vi "Format CSV.vi"(8 "error in (no error)":errorcluster, 9 "delimiter":string=",", 10 "CSV File Input":path, 11 "Original CSV Format":enum16{"Format A", "Format B"}(ring)) -> (0 "error out":errorcluster, 1 "Parcel Length":i32[](array[numeric]), 2 "All Terminal Data":T1(array[cluster]))   [LabVIEW 2017] (continued)
"28:39.7", "28:39.8", "28:39.8", "28:39.8", "28:39.9", "28:39.9", "28:39.9", "28:40.0", "28:40.0", "28:40.0", "28:40.1", "28:40.1", "28:40.1", "28:40.2", "28:40.2", "28:40.2", "28:40.3", "28:40.3", "28:40.3", "28:40.4", "28:40.4", "28:40.4", "28:40.5", "28:40.5", "28:40.5", "28:40.6", "28:40.6", "28:40.6", "28:40.7", "28:40.7", "28:40.7", "28:40.8", "28:40.8", "28:40.8", "28:40.9", "28:40.9", "28:40.9", "28:41.0", "28:41.0", "28:41.0", "28:41.1", "28:41.1", "28:41.1", "28:41.2", "28:41.2", "28:41.2", "28:41.3", "28:41.3", "28:41.3", "28:41.4", "28:41.4", "28:41.4", "28:41.5", "28:41.5", "28:41.5", "28:41.6", "28:41.6", "28:41.6", "28:41.7", "28:41.7", "28:41.7", "28:41.8", "28:41.8", "28:41.8", "28:41.9", "28:41.9", "28:41.9", "28:42.0", "28:42.0", "28:42.0", "28:42.1", "28:42.1", "28:42.1", "28:42.2", "28:42.2", "28:42.2", "28:42.3", "28:42.3", "28:42.3", "28:42.4", "28:42.4", "28:42.4", "28:42.5", "28:42.5", "28:42.5", "28:42.6", "28:42.6", "28:42.6", "28:42.7", "28:42.7", "28:42.7", "28:42.8", "28:42.8", "28:42.8", "28:42.9", "28:42.9", "28:42.9", "28:43.0", "28:43.0", "28:43.0", "28:43.1", "28:43.1", "28:43.1", "28:43.2", "28:43.2", "28:43.2", "28:43.3", "28:43.3", "28:43.3", "28:43.4", "28:43.4", "28:43.4", "28:43.5", "28:43.5", "28:43.5", "28:43.6", "28:43.6", "28:43.6", "28:43.7", "28:43.7", "28:43.7", "28:43.8", "28:43.8", "28:43.8", "28:43.9", "28:43.9", "28:43.9", "28:44.0", "28:44.0", "28:44.0", "28:44.1", "28:44.1", "28:44.1", "28:44.2", "28:44.2", "28:44.2", "28:44.3", "28:44.3", "28:44.3", "28:44.4", "28:44.4", "28:44.4", "28:44.5", "28:44.5", "28:44.5", "28:44.6", "28:44.6", "28:44.6", "28:44.7", "28:44.7", "28:44.7", "28:44.8", "28:44.8", "28:44.8", "28:44.9", "28:44.9", "28:44.9", "28:45.0", "28:45.0", "28:45.0", "28:45.1", "28:45.1", "28:45.1", "28:45.2", "28:45.2", "28:45.2", "28:45.3", "28:45.3", "28:45.3", "28:45.4", "28:45.4", "28:45.4", "28:45.5", "28:45.5", "28:45.5", "28:45.6", "28:45.6", "28:45.6", "28:45.7", "28:45.7", "28:45.7", "28:45.8", "28:45.8", "28:45.8", "28:45.9", "28:45.9", "28:45.9", "28:46.0", "28:46.0", "28:46.0", "28:46.1", "28:46.1", "28:46.1", "28:46.2", "28:46.2", "28:46.2", "28:46.3", "28:46.3", "28:46.3", "28:46.4", "28:46.4", "28:46.4", "28:46.5", "28:46.5", "28:46.5", "28:46.6", "28:46.6", "28:46.6", "28:46.7", "28:46.7", "28:46.7", "28:46.8", "28:46.8", "28:46.8", "28:46.9", "28:46.9", "28:46.9", "28:47.0", "28:47.0", "28:47.0", "28:47.1", "28:47.1", "28:47.1", "28:47.2", "28:47.2", "28:47.2", "28:47.3", "28:47.3", "28:47.3", "28:47.4", "28:47.4", "28:47.4", "28:47.5", "28:47.5", "28:47.5", "28:47.6", "28:47.6", "28:47.6", "28:47.7", "28:47.7", "28:47.7", "28:47.8", "28:47.8", "28:47.8", "28:47.9", "28:47.9", "28:47.9", "28:48.0", "28:48.0", "28:48.0", "28:48.1", "28:48.1", "28:48.1", "28:48.2", "28:48.2", "28:48.2", "28:48.3", "28:48.3", "28:48.3", "28:48.4", "28:48.4", "28:48.4", "28:48.5", "28:48.5", "28:48.5", "28:48.6", "28:48.6", "28:48.6", "28:48.7", "28:48.7", "28:48.7", "28:48.8", "28:48.8", "28:48.8", "28:48.9", "28:48.9", "28:48.9", "28:49.0", "28:49.0", "28:49.0", "28:49.1", "28:49.1", "28:49.1", "28:49.2", "28:49.2", "28:49.2", "28:49.3", "28:49.3", "28:49.3", "28:49.4", "28:49.4", "28:49.4", "28:49.5", "28:49.5", "28:49.5", "28:49.6", "28:49.6", "28:49.6", "28:49.7", "28:49.7", "28:49.7", "28:49.8", "28:49.8", "28:49.8", "28:49.9", "28:49.9", "28:49.9", "28:50.0", "28:50.0", "28:50.0", "28:50.1", "28:50.1", "28:50.1", "28:50.2", "28:50.2", "28:50.2", "28:50.3", "28:50.3", "28:50.3", "28:50.4", "28:50.4", "28:50.4", "28:50.5", "28:50.5", "28:50.5", "28:50.6", "28:50.6", "28:50.6", "28:50.7", "28:50.7", "28:50.7", "28:50.8", "28:50.8", "28:50.8", "28:50.9", "28:50.9", "28:50.9", "28:51.0", "28:51.0", "28:51.0", "28:51.1", "28:51.1", "28:51.1", "28:51.2", "28:51.2", "28:51.2", "28:51.3", "28:51.3", "28:51.3", "28:51.4", "28:51.4", "28:51.4", "28:51.5", "28:51.5", "28:51.5", "28:51.6", "28:51.6", "28:51.6", "28:51.7", "28:51.7", "28:51.7", "28:51.8", "28:51.8", "28:51.8", "28:51.9", "28:51.9", "28:51.9", "28:52.0", "28:52.0", "28:52.0", "28:52.1", "28:52.1", "28:52.1", "28:52.2", "28:52.2", "28:52.2", "28:52.3", "28:52.3", "28:52.3", "28:52.4", "28:52.4", "28:52.4", "28:52.5", "28:52.5", "28:52.5", "28:52.6", "28:52.6", "28:52.6", "28:52.7", "28:52.7", "28:52.7", "28:52.8", "28:52.8", "28:52.8", "28:52.9", "28:52.9", "28:52.9", "28:53.0", "28:53.0", "28:53.0", "28:53.1", "28:53.1", "28:53.1", "28:53.2", "28:53.2", "28:53.2", "28:53.3", "28:53.3", "28:53.3", "28:53.4", "28:53.4", "28:53.4", "28:53.5", "28:53.5", "28:53.5", "28:53.6", "28:53.6", "28:53.6", "28:53.7", "28:53.7", "28:53.7", "28:53.8", "28:53.8", "28:53.8", "28:53.9", "28:53.9", "28:53.9", "28:54.0", "28:54.0", "28:54.0", "28:54.1", "28:54.1", "28:54.1", "28:54.2", "28:54.2", "28:54.2", "28:54.3", "28:54.3", "28:54.3", "28:54.4", "28:54.4", "28:54.4", "28:54.5", "28:54.5", "28:54.5", "28:54.6", "28:54.6", "28:54.6", "28:54.7", "28:54.7", "28:54.7", "28:54.8", "28:54.8", "28:54.8", "28:54.9", "28:54.9", "28:54.9", "28:55.0", "28:55.0", "28:55.0", "28:55.1", "28:55.1", "28:55.1", "28:55.2", "28:55.2", "28:55.2", "28:55.3", "28:55.3", "28:55.3", "28:55.4", "28:55.4", "28:55.4", "28:55.5", "28:55.5", "28:55.5", "28:55.6", "28:55.6", "28:55.6", "28:55.7", "28:55.7", "28:55.7", "28:55.8", "28:55.8", "28:55.8", "28:55.9", "28:55.9", "28:55.9", "28:56.0", "28:56.0", "28:56.0", "28:56.1", "28:56.1", "28:56.1", "28:56.2", "28:56.2", "28:56.2", "28:56.3", "28:56.3", "28:56.3", "28:56.4", "28:56.4", "28:56.4", "28:56.5", "28:56.5", "28:56.5", "28:56.6", "28:56.6", "28:56.6", "28:56.7", "28:56.7", "28:56.7", "28:56.8", "28:56.8", "28:56.8", "28:56.9", "28:56.9", "28:56.9", "28:57.0", "28:57.0", "28:57.0", "28:57.1", "28:57.1", "28:57.1", "28:57.2", "28:57.2", "28:57.2", "28:57.3", "28:57.3", "28:57.3", "28:57.4", "28:57.4", "28:57.4", "28:57.5", "28:57.5", "28:57.5", "28:57.6", "28:57.6", "28:57.6", "28:57.7", "28:57.7", "28:57.7", "28:57.8", "28:57.8", "28:57.8", "28:57.9", "28:57.9", "28:57.9", "28:58.0", "28:58.0", "28:58.0", "28:58.1", "28:58.1", "28:58.1", "28:58.2", "28:58.2", "28:58.2", "28:58.3", "28:58.3", "28:58.3", "28:58.4", "28:58.4", "28:58.4", "28:58.5", "28:58.5", "28:58.5", "28:58.6", "28:58.6", "28:58.6", "28:58.7", "28:58.7", "28:58.7", "28:58.8", "28:58.8", "28:58.8", "28:58.9", "28:58.9", "28:58.9", "28:59.0", "28:59.0", "28:59.0", "28:59.1", "28:59.1", "28:59.1", "28:59.2", "28:59.2", "28:59.2", "28:59.3", "28:59.3", "28:59.3", "28:59.4", "28:59.4", "28:59.4", "28:59.5", "28:59.5", "28:59.5", "28:59.6", "28:59.6", "28:59.6", "28:59.7", "28:59.7", "28:59.7", "28:59.8", "28:59.8", "28:59.8", "28:59.9", "28:59.9", "28:59.9", "29:00.0", "29:00.0", "29:00.0", "29:00.1", "29:00.1", "29:00.1", "29:00.2", "29:00.2", "29:00.2", "29:00.3", "29:00.3", "29:00.3", "29:00.4", "29:00.4", "29:00.4", "29:00.5", "29:00.5", "29:00.5", "29:00.6", "29:00.6", "29:00.6", "29:00.7", "29:00.7", "29:00.7", "29:00.8", "29:00.8", "29:00.8", "29:00.9", "29:00.9", "29:00.9", "29:01.0", "29:01.0", "29:01.0", "29:01.1", "29:01.1", "29:01.1", "29:01.2", "29:01.2", "29:01.2", "29:01.3", "29:01.3", "29:01.3", "29:01.4", "29:01.4", "29:01.4", "29:01.5", "29:01.5", "29:01.5", "29:01.6", "29:01.6", "29:01.6", "29:01.7", "29:01.7", "29:01.7", "29:01.8", "29:01.8", "29:01.8", "29:01.9", "29:01.9", "29:01.9", "29:02.0", "29:02.0", "29:02.0", "29:02.1", "29:02.1", "29:02.1", "29:02.2", "29:02.2", "29:02.2", "29:02.3", "29:02.3", "29:02.3", "29:02.4", "29:02.4", "29:02.4", "29:02.5", "29:02.5", "29:02.5", "29:02.6", "29:02.6", "29:02.6", "29:02.7", "29:02.7", "29:02.7", "29:02.8", "29:02.8", "29:02.8", "29:02.9", "29:02.9", "29:02.9", "29:03.0", "29:03.0", "29:03.0", "29:03.1", "29:03.1", "29:03.1", "29:03.2", "29:03.2", "29:03.2", "29:03.3", "29:03.3", "29:03.3", "29:03.4", "29:03.4", "29:03.4", "29:03.5", "29:03.5", "29:03.5", "29:03.6", "29:03.6", "29:03.6", "29:03.7", "29:03.7", "29:03.7", "29:03.8", "29:03.8", "29:03.8", "29:03.9", "29:03.9", "29:03.9", "29:04.0", "29:04.0", "29:04.0", "29:04.1", "29:04.1", "29:04.1", "29:04.2", "29:04.2", "29:04.2", "29:04.3", "29:04.3", "29:04.3", "29:04.4", "29:04.4", "29:04.4", "29:04.5", "29:04.5", "29:04.5", "29:04.6", "29:04.6", "29:04.6", "29:04.7", "29:04.7", "29:04.7", "29:04.8", "29:04.8", "29:04.8", "29:04.9", "29:04.9", "29:04.9", "29:05.0", "29:05.0", "29:05.0", "29:05.1", "29:05.1", "29:05.1", "29:05.2", "29:05.2", "29:05.2", "29:05.3", "29:05.3", "29:05.3", "29:05.4", "29:05.4", "29:05.4", "29:05.5", "29:05.5", "29:05.5", "29:05.6", "29:05.6", "29:05.6", "29:05.7", "29:05.7", "29:05.7", "29:05.8", "29:05.8", "29:05.8", "29:05.9", "29:05.9", "29:05.9", "29:06.0", "29:06.0", "29:06.0", "29:06.1", "29:06.1", "29:06.1", "29:06.2", "29:06.2", "29:06.2", "29:06.3", "29:06.3", "29:06.3", "29:06.4", "29:06.4", "29:06.4", "29:06.5", "29:06.5", "29:06.5", "29:06.6", "29:06.6", "29:06.6", "29:06.7", "29:06.7", "29:06.7", "29:06.8", "29:06.8", "29:06.8", "29:06.9", "29:06.9", "29:06.9", "29:07.0", "29:07.0", "29:07.0", "29:07.1", "29:07.1", "29:07.1", "29:07.2", "29:07.2", "29:07.2", "29:07.3", "29:07.3", "29:07.3", "29:07.4", "29:07.4", "29:07.4", "29:07.5", "29:07.5", "29:07.5", "29:07.6", "29:07.6", "29:07.6", "29:07.7", "29:07.7", "29:07.7", "29:07.8", "29:07.8", "29:07.8", "29:07.9", "29:07.9", "29:07.9", "29:08.0", "29:08.0", "29:08.0", "29:08.1", "29:08.1", "29:08.1", "29:08.2", "29:08.2", "29:08.2", "29:08.3", "29:08.3", "29:08.3", "29:08.4", "29:08.4", "29:08.4", "29:08.5", "29:08.5", "29:08.5", "29:08.6", "29:08.6", "29:08.6", "29:08.7", "29:08.7", "29:08.7", "29:08.8", "29:08.8", "29:08.8", "29:08.9", "29:08.9", "29:08.9", "29:09.0", "29:09.0", "29:09.0", "29:09.1", "29:09.1", "29:09.1", "29:09.2", "29:09.2", "29:09.2", "29:09.3", "29:09.3", "29:09.3", "29:09.4", "29:09.4", "29:09.4", "29:09.5", "29:09.5", "29:09.5", "29:09.6", "29:09.6", "29:09.6", "29:09.7", "29:09.7", "29:09.7", "29:09.8", "29:09.8", "29:09.8", "29:09.9", "29:09.9", "29:09.9", "29:10.0", "29:10.0", "29:10.0", "29:10.1", "29:10.1", "29:10.1", "29:10.2", "29:10.2", "29:10.2", "29:10.3", "29:10.3", "29:10.3", "29:10.4", "29:10.4", "29:10.4", "29:10.5", "29:10.5", "29:10.5", "29:10.6", "29:10.6", "29:10.6", "29:10.7", "29:10.7", "29:10.7", "29:10.8", "29:10.8", "29:10.8", "29:10.9", "29:10.9", "29:10.9", "29:11.0", "29:11.0", "29:11.0", "29:11.1", "29:11.1", "29:11.1", "29:11.2", "29:11.2", "29:11.2", "29:11.3", "29:11.3", "29:11.3", "29:11.4", "29:11.4", "29:11.4", "29:11.5", "29:11.5", "29:11.5", "29:11.6", "29:11.6", "29:11.6", "29:11.7", "29:11.7", "29:11.7", "29:11.8", "29:11.8", "29:11.8", "29:11.9", "29:11.9", "29:11.9", "29:12.0", "29:12.0", "29:12.0", "29:12.1", "29:12.1", "29:12.1", "29:12.2", "29:12.2", "29:12.2", "29:12.3", "29:12.3", "29:12.3", "29:12.4", "29:12.4", "29:12.4", "29:12.5", "29:12.5", "29:12.5", "29:12.6", "29:12.6", "29:12.6", "29:12.7", "29:12.7", "29:12.7", "29:12.8", "29:12.8", "29:12.8", "29:12.9", "29:12.9", "29:12.9", "29:13.0", "29:13.0", "29:13.0", "29:13.1", "29:13.1", "29:13.1", "29:13.2", "29:13.2", "29:13.2", "29:13.3", "29:13.3", "29:13.3", "29:13.4", "29:13.4", "29:13.4", "29:13.5", "29:13.5", "29:13.5", "29:13.6", "29:13.6", "29:13.6", "29:13.7", "29:13.7", "29:13.7", "29:13.8", "29:13.8", "29:13.8", "29:13.9", "29:13.9", "29:13.9", "29:14.0", "29:14.0", "29:14.0", "29:14.1", "29:14.1", "29:14.1", "29:14.2", "29:14.2", "29:14.2", "29:14.3", "29:14.3", "29:14.3", "29:14.4", "29:14.4", "29:14.4", "29:14.5", "29:14.5", "29:14.5", "29:14.6", "29:14.6", "29:14.6", "29:14.7", "29:14.7", "29:14.7", "29:14.8", "29:14.8", "29:14.8", "29:14.9", "29:14.9", "29:14.9", "29:15.0", "29:15.0", "29:15.0", "29:15.1", "29:15.1", "29:15.1", "29:15.2", "29:15.2", "29:15.2", "29:15.3", "29:15.3", "29:15.3", "29:15.4", "29:15.4", "29:15.4", "29:15.5", "29:15.5", "29:15.5", "29:15.6", "29:15.6", "29:15.6", "29:15.7", "29:15.7", "29:15.7", "29:15.8", "29:15.8", "29:15.8", "29:15.9", "29:15.9", "29:15.9", "29:16.0", "29:16.0", "29:16.0", "29:16.1", "29:16.1", "29:16.1", "29:16.2", "29:16.2", "29:16.2", "29:16.3", "29:16.3", "29:16.3", "29:16.4", "29:16.4", "29:16.4", "29:16.5", "29:16.5", "29:16.5", "29:16.6", "29:16.6", "29:16.6", "29:16.7", "29:16.7", "29:16.7", "29:16.8", "29:16.8", "29:16.8", "29:16.9", "29:16.9", "29:16.9", "29:17.0", "29:17.0", "29:17.0", "29:17.1", "29:17.1", "29:17.1", "29:17.2", "29:17.2", "29:17.2", "29:17.3", "29:17.3", "29:17.3", "29:17.4", "29:17.4", "29:17.4", "29:17.5", "29:17.5", "29:17.5", "29:17.6", "29:17.6", "29:17.6", "29:17.7", "29:17.7", "29:17.7", "29:17.8", "29:17.8", "29:17.8", "29:17.9", "29:17.9", "29:17.9", "29:18.0", "29:18.0", "29:18.0", "29:18.1", "29:18.1", "29:18.1", "29:18.2", "29:18.2", "29:18.2", "29:18.3", "29:18.3", "29:18.3", "29:18.4", "29:18.4", "29:18.4", "29:18.5", "29:18.5", "29:18.5", "29:18.6", "29:18.6", "29:18.6", "29:18.7", "29:18.7", "29:18.7", "29:18.8", "29:18.8", "29:18.8", "29:18.9", "29:18.9", "29:18.9", "29:19.0", "29:19.0", "29:19.0", "29:19.1", "29:19.1", "29:19.1", "29:19.2", "29:19.2", "29:19.2", "29:19.3", "29:19.3", "29:19.3", "29:19.4", "29:19.4", "29:19.4", "29:19.5", "29:19.5", "29:19.5", "29:19.6", "29:19.6", "29:19.6", "29:19.7", "29:19.7", "29:19.7", "29:19.8", "29:19.8", "29:19.8", "29:19.9", "29:19.9", "29:19.9", "29:20.0", "29:20.0", "29:20.0", "29:20.1", "29:20.1", "29:20.1", "29:20.2", "29:20.2", "29:20.2", "29:20.3", "29:20.3", "29:20.3", "29:20.4", "29:20.4", "29:20.4", "29:20.5", "29:20.5", "29:20.5", "29:20.6", "29:20.6", "29:20.6", "29:20.7", "29:20.7", "29:20.7", "29:20.8", "29:20.8", "29:20.8", "29:20.9", "29:20.9", "29:20.9", "29:21.0", "29:21.0", "29:21.0", "29:21.1", "29:21.1", "29:21.1", "29:21.2", "29:21.2", "29:21.2", "29:21.3", "29:21.3", "29:21.3", "29:21.4", "29:21.4", "29:21.4", "29:21.5", "29:21.5", "29:21.5", "29:21.6", "29:21.6", "29:21.6", "29:21.7", "29:21.7", "29:21.7", "29:21.8", "29:21.8", "29:21.8", "29:21.9", "29:21.9", "29:21.9", "29:22.0", "29:22.0", "29:22.0", "29:22.1", "29:22.1", "29:22.1", "29:22.2", "29:22.2", "29:22.2", "29:22.3", "29:22.3", "29:22.3", "29:22.4", "29:22.4", "29:22.4", "29:22.5", "29:22.5", "29:22.5", "29:22.6", "29:22.6", "29:22.6", "29:22.7", "29:22.7", "29:22.7", "29:22.8", "29:22.8", "29:22.8", "29:22.9", "29:22.9", "29:22.9", "29:23.0", "29:23.0", "29:23.0", "29:23.1", "29:23.1", "29:23.1", "29:23.2", "29:23.2", "29:23.2", "29:23.3", "29:23.3", "29:23.3", "29:23.4", "29:23.4", "29:23.4", "29:23.5", "29:23.5", "29:23.5", "29:23.6", "29:23.6", "29:23.6", "29:23.7", "29:23.7", "29:23.7", "29:23.8", "29:23.8", "29:23.8", "29:23.9", "29:23.9", "29:23.9", "29:24.0", "29:24.0", "29:24.0", "29:24.1", "29:24.1", "29:24.1", "29:24.2", "29:24.2", "29:24.2", "29:24.3", "29:24.3", "29:24.3", "29:24.4", "29:24.4", "29:24.4", "29:24.5", "29:24.5", "29:24.5", "29:24.6", "29:24.6", "29:24.6", "29:24.7", "29:24.7", "29:24.7", "29:24.8", "29:24.8", "29:24.8", "29:24.9", "29:24.9", "29:24.9", "29:25.0", "29:25.0", "29:25.0", "29:25.1", "29:25.1", "29:25.1", "29:25.2", "29:25.2", "29:25.2", "29:25.3", "29:25.3", "29:25.3", "29:25.4", "29:25.4", "29:25.4", "29:25.5", "29:25.5", "29:25.5", "29:25.6", "29:25.6", "29:25.6", "29:25.7", "29:25.7", "29:25.7", "29:25.8", "29:25.8", "29:25.8", "29:25.9", "29:25.9", "29:25.9", "29:26.0", "29:26.0", "29:26.0", "29:26.1", "29:26.1", "29:26.1", "29:26.2", "29:26.2", "29:26.2", "29:26.3", "29:26.3", "29:26.3", "29:26.4", "29:26.4", "29:26.4", "29:26.5", "29:26.5", "29:26.5", "29:26.6", "29:26.6", "29:26.6", "29:26.7", "29:26.7", "29:26.7", "29:26.8", "29:26.8", "29:26.8", "29:26.9", "29:26.9", "29:26.9", "29:27.0", "29:27.0", "29:27.0", "29:27.1", "29:27.1", "29:27.1", "29:27.2", "29:27.2", "29:27.2", "29:27.3", "29:27.3", "29:27.3", "29:27.4", "29:27.4", "29:27.4", "29:27.5", "29:27.5", "29:27.5", "29:27.6", "29:27.6", "29:27.6", "29:27.7", "29:27.7", "29:27.7", "29:27.8", "29:27.8", "29:27.8", "29:27.9", "29:27.9", "29:27.9", "29:28.0", "29:28.0", "29:28.0", "29:28.1", "29:28.1", "29:28.1", "29:28.2", "29:28.2", "29:28.2", "29:28.3", "29:28.3", "29:28.3", "29:28.4", "29:28.4", "29:28.4", "29:28.5", "29:28.5", "29:28.5", "29:28.6", "29:28.6", "29:28.6", "29:28.7", "29:28.7", "29:28.7", "29:28.8", "29:28.8", "29:28.8", "29:28.9", "29:28.9", "29:28.9", "29:29.0", "29:29.0", "29:29.0", "29:29.1", "29:29.1", "29:29.1", "29:29.2", "29:29.2", "29:29.2", "29:29.3", "29:29.3", "29:29.3", "29:29.4", "29:29.4", "29:29.4", "29:29.5", "29:29.5", "29:29.5", "29:29.6", "29:29.6", "29:29.6", "29:29.7", "29:29.7", "29:29.7", "29:29.8", "29:29.8", "29:29.8", "29:29.9", "29:29.9", "29:29.9", "29:30.0", "29:30.0", "29:30.0", "29:30.1", "29:30.1", "29:30.1", "29:30.2", "29:30.2", "29:30.2", "29:30.3", "29:30.3", "29:30.3", "29:30.4", "29:30.4", "29:30.4", "29:30.5", "29:30.5", "29:30.5", "29:30.6", "29:30.6", "29:30.6", "29:30.7", "29:30.7", "29:30.7", "29:30.8", "29:30.8", "29:30.8", "29:30.9", "29:30.9", "29:30.9", "29:31.0", "29:31.0", "29:31.0", "29:31.1", "29:31.1", "29:31.1", "29:31.2", "29:31.2", "29:31.2", "29:31.3", "29:31.3", "29:31.3", "29:31.4", "29:31.4", "29:31.4", "29:31.5", "29:31.5", "29:31.5", "29:31.6", "29:31.6", "29:31.6", "29:31.7", "29:31.7", "29:31.7", "29:31.8", "29:31.8", "29:31.8", "29:31.9", "29:31.9", "29:31.9", "29:32.0", "29:32.0", "29:32.0", "29:32.1", "29:32.1", "29:32.1", "29:32.2", "29:32.2", "29:32.2", "29:32.3", "29:32.3", "29:32.3", "29:32.4", "29:32.4", "29:32.4", "29:32.5", "29:32.5", "29:32.5", "29:32.6", "29:32.6", "29:32.6", "29:32.7", "29:32.7", "29:32.7", "29:32.8", "29:32.8", "29:32.8", "29:32.9", "29:32.9", "29:32.9", "29:33.0", "29:33.0", "29:33.0", "29:33.1", "29:33.1", "29:33.1", "29:33.2", "29:33.2", "29:33.2", "29:33.3", "29:33.3", "29:33.3", "29:33.4", "29:33.4", "29:33.4", "29:33.5", "29:33.5", "29:33.5", "29:33.6", "29:33.6", "29:33.6", "29:33.7", "29:33.7", "29:33.7", "29:33.8", "29:33.8", "29:33.8", "29:33.9", "29:33.9", "29:33.9", "29:34.0", "29:34.0", "29:34.0", "29:34.1", "29:34.1", "29:34.1", "29:34.2", "29:34.2", "29:34.2", "29:34.3", "29:34.3", "29:34.3", "29:34.4", "29:34.4", "29:34.4", "29:34.5", "29:34.5", "29:34.5", "29:34.6", "29:34.6", "29:34.6", "29:34.7", "29:34.7", "29:34.7", "29:34.8", "29:34.8", "29:34.8", "29:34.9", "29:34.9", "29:34.9", "29:35.0", "29:35.0", "29:35.0", "29:35.1", "29:35.1", "29:35.1", "29:35.2", "29:35.2", "29:35.2", "29:35.3", "29:35.3", "29:35.3", "29:35.4", "29:35.4", "29:35.4", "29:35.5", "29:35.5", "29:35.5", "29:35.6", "29:35.6", "29:35.6", "29:35.7", "29:35.7", "29:35.7", "29:35.8", "29:35.8", "29:35.8", "29:35.9", "29:35.9", "29:35.9", "29:36.0", "29:36.0", "29:36.0", "29:36.1", "29:36.1", "29:36.1", "29:36.2", "29:36.2", "29:36.2", "29:36.3", "29:36.3", "29:36.3", "29:36.4", "29:36.4", "29:36.4", "29:36.5", "29:36.5", "29:36.5", "29:36.6", "29:36.6", "29:36.6", "29:36.7", "29:36.7", "29:36.7", "29:36.8", "29:36.8", "29:36.8", "29:36.9", "29:36.9", "29:36.9", "29:37.0", "29:37.0", "29:37.0", "29:37.1", "29:37.1", "29:37.1", "29:37.2", "29:37.2", "29:37.2", "29:37.3", "29:37.3", "29:37.3", "29:37.4", "29:37.4", "29:37.4", "29:37.5", "29:37.5", "29:37.5", "29:37.6", "29:37.6", "29:37.6", "29:37.7", "29:37.7", "29:37.7", "29:37.8", "29:37.8", "29:37.8", "29:37.9", "29:37.9", "29:37.9", "29:38.0", "29:38.0", "29:38.0", "29:38.1", "29:38.1", "29:38.1", "29:38.2", "29:38.2", "29:38.2", "29:38.3", "29:38.3", "29:38.3", "29:38.4", "29:38.4", "29:38.4", "29:38.5", "29:38.5", "29:38.5", "29:38.6", "29:38.6", "29:38.6", "29:38.7", "29:38.7", "29:38.7", "29:38.8", "29:38.8", "29:38.8", "29:38.9", "29:38.9", "29:38.9", "29:39.0", "29:39.0", "29:39.0", "29:39.1", "29:39.1", "29:39.1", "29:39.2", "29:39.2", "29:39.2", "29:39.3", "29:39.3", "29:39.3", "29:39.4", "29:39.4", "29:39.4", "29:39.5", "29:39.5", "29:39.5", "29:39.6", "29:39.6", "29:39.6", "29:39.7", "29:39.7", "29:39.7", "29:39.8", "29:39.8", "29:39.8", "29:39.9", "29:39.9", "29:39.9", "29:40.0", "29:40.0", "29:40.0", "29:40.1", "29:40.1", "29:40.1", "29:40.2", "29:40.2", "29:40.2", "29:40.3", "29:40.3", "29:40.3", "29:40.4", "29:40.4", "29:40.4", "29:40.5", "29:40.5", "29:40.5", "29:40.6", "29:40.6", "29:40.6", "29:40.7", "29:40.7", "29:40.7", "29:40.8", "29:40.8", "29:40.8", "29:40.9", "29:40.9", "29:40.9", "29:41.0", "29:41.0", "29:41.0", "29:41.1", "29:41.1", "29:41.1", "29:41.2", "29:41.2", "29:41.2", "29:41.3", "29:41.3", "29:41.3", "29:41.4", "29:41.4", "29:41.4", "29:41.5", "29:41.5", "29:41.5", "29:41.6", "29:41.6", "29:41.6", "29:41.7", "29:41.7", "29:41.7", "29:41.8", "29:41.8", "29:41.8", "29:41.9", "29:41.9", "29:41.9", "29:42.0", "29:42.0", "29:42.0", "29:42.1", "29:42.1", "29:42.1", "29:42.2", "29:42.2", "29:42.2", "29:42.3", "29:42.3", "29:42.3", "29:42.4", "29:42.4", "29:42.4", "29:42.5", "29:42.5", "29:42.5", "29:42.6", "29:42.6", "29:42.6", "29:42.7", "29:42.7", "29:42.7", "29:42.8", "29:42.8", "29:42.8", "29:42.9", "29:42.9", "29:42.9", "29:43.0", "29:43.0", "29:43.0", "29:43.1", "29:43.1", "29:43.1", "29:43.2", "29:43.2", "29:43.2", "29:43.3", "29:43.3", "29:43.3", "29:43.4", "29:43.4", "29:43.4", "29:43.5", "29:43.5", "29:43.5", "29:43.6", "29:43.6", "29:43.6", "29:43.7", "29:43.7", "29:43.7", "29:43.8", "29:43.8", "29:43.8", "29:43.9", "29:43.9", "29:43.9", "29:44.0", "29:44.0", "29:44.0", "29:44.1", "29:44.1", "29:44.1", "29:44.2", "29:44.2", "29:44.2", "29:44.3", "29:44.3", "29:44.3", "29:44.4", "29:44.4", "29:44.4", "29:44.5", "29:44.5", "29:44.5", "29:44.6", "29:44.6", "29:44.6", "29:44.7", "29:44.7", "29:44.7", "29:44.8", "29:44.8", "29:44.8", "29:44.9", "29:44.9", "29:44.9", "29:45.0", "29:45.0", "29:45.0", "29:45.1", "29:45.1", "29:45.1", "29:45.2", "29:45.2", "29:45.2", "29:45.3", "29:45.3", "29:45.3", "29:45.4", "29:45.4", "29:45.4", "29:45.5", "29:45.5", "29:45.5", "29:45.6", "29:45.6", "29:45.6", "29:45.7", "29:45.7", "29:45.7", "29:45.8", "29:45.8", "29:45.8", "29:45.9", "29:45.9", "29:45.9", "29:46.0", "29:46.0", "29:46.0", "29:46.1", "29:46.1", "29:46.1", "29:46.2", "29:46.2", "29:46.2", "29:46.3", "29:46.3", "29:46.3", "29:46.4", "29:46.4", "29:46.4", "29:46.5", "29:46.5", "29:46.5", "29:46.6", "29:46.6", "29:46.6", "29:46.7", "29:46.7", "29:46.7", "29:46.8", "29:46.8", "29:46.8", "29:46.9", "29:46.9", "29:46.9", "29:47.0", "29:47.0", "29:47.0", "29:47.1", "29:47.1", "29:47.1", "29:47.2", "29:47.2", "29:47.2", "29:47.3", "29:47.3", "29:47.3", "29:47.4", "29:47.4", "29:47.4", "29:47.5", "29:47.5", "29:47.5", "29:47.6", "29:47.6", "29:47.6", "29:47.7", "29:47.7", "29:47.7", "29:47.8", "29:47.8", "29:47.8", "29:47.9", "29:47.9", "29:47.9", "29:48.0", "29:48.0", "29:48.0", "29:48.1", "29:48.1", "29:48.1", "29:48.2", "29:48.2", "29:48.2", "29:48.3", "29:48.3", "29:48.3", "29:48.4", "29:48.4", "29:48.4", "29:48.5", "29:48.5", "29:48.5", "29:48.6", "29:48.6", "29:48.6", "29:48.7", "29:48.7", "29:48.7", "29:48.8", "29:48.8", "29:48.8", "29:48.9", "29:48.9", "29:48.9", "29:49.0", "29:49.0", "29:49.0", "29:49.1", "29:49.1", "29:49.1", "29:49.2", "29:49.2", "29:49.2", "29:49.3", "29:49.3", "29:49.3", "29:49.4", "29:49.4", "29:49.4", "29:49.5", "29:49.5", "29:49.5", "29:49.6", "29:49.6", "29:49.6", "29:49.7", "29:49.7", "29:49.7", "29:49.8", "29:49.8", "29:49.8", "29:49.9", "29:49.9", "29:49.9", "29:50.0", "29:50.0", "29:50.0", "29:50.1", "29:50.1", "29:50.1", "29:50.2", "29:50.2", "29:50.2", "29:50.3", "29:50.3", "29:50.3", "29:50.4", "29:50.4", "29:50.4", "29:50.5", "29:50.5", "29:50.5", "29:50.6", "29:50.6", "29:50.6", "29:50.7", "29:50.7", "29:50.7", "29:50.8", "29:50.8", "29:50.8", "29:50.9", "29:50.9", "29:50.9", "29:51.0", "29:51.0", "29:51.0", "29:51.1", "29:51.1", "29:51.1", "29:51.2", "29:51.2", "29:51.2", "29:51.3", "29:51.3", "29:51.3", "29:51.4", "29:51.4", "29:51.4", "29:51.5", "29:51.5", "29:51.5", "29:51.6", "29:51.6", "29:51.6", "29:51.7", "29:51.7", "29:51.7", "29:51.8", "29:51.8", "29:51.8", "29:51.9", "29:51.9", "29:51.9", "29:52.0", "29:52.0", "29:52.0", "29:52.1", "29:52.1", "29:52.1", "29:52.2", "29:52.2", "29:52.2", "29:52.3", "29:52.3", "29:52.3", "29:52.4", "29:52.4", "29:52.4", "29:52.5", "29:52.5", "29:52.5", "29:52.6", "29:52.6", "29:52.6", "29:52.7", "29:52.7", "29:52.7", "29:52.8", "29:52.8", "29:52.8", "29:52.9", "29:52.9", "29:52.9", "29:53.0", "29:53.0", "29:53.0", "29:53.1", "29:53.1", "29:53.1", "29:53.2", "29:53.2", "29:53.2", "29:53.3", "29:53.3", "29:53.3", "29:53.4", "29:53.4", "29:53.4", "29:53.5", "29:53.5", "29:53.5", "29:53.6", "29:53.6", "29:53.6", "29:53.7", "29:53.7", "29:53.7", "29:53.8", "29:53.8", "29:53.8", "29:53.9", "29:53.9", "29:53.9", "29:54.0", "29:54.0", "29:54.0", "29:54.1", "29:54.1", "29:54.1", "29:54.2", "29:54.2", "29:54.2", "29:54.3", "29:54.3", "29:54.3", "29:54.4", "29:54.4", "29:54.4", "29:54.5", "29:54.5", "29:54.5", "29:54.6", "29:54.6", "29:54.6", "29:54.7", "29:54.7", "29:54.7", "29:54.8", "29:54.8", "29:54.8", "29:54.9", "29:54.9", "29:54.9", "29:55.0", "29:55.0", "29:55.0", "29:55.1", "29:55.1", "29:55.1", "29:55.2", "29:55.2", "29:55.2", "29:55.3", "29:55.3", "29:55.3", "29:55.4", "29:55.4", "29:55.4", "29:55.5", "29:55.5", "29:55.5", "29:55.6", "29:55.6", "29:55.6", "29:55.7", "29:55.7", "29:55.7", "29:55.8", "29:55.8", "29:55.8", "29:55.9", "29:55.9", "29:55.9", "29:56.0", "29:56.0", "29:56.0", "29:56.1", "29:56.1", "29:56.1", "29:56.2", "29:56.2", "29:56.2", "29:56.3", "29:56.3", "29:56.3", "29:56.4", "29:56.4", "29:56.4", "29:56.5", "29:56.5", "29:56.5", "29:56.6", "29:56.6", "29:56.6", "29:56.7", "29:56.7", "29:56.7", "29:56.8", "29:56.8", "29:56.8", "29:56.9", "29:56.9", "29:56.9", "29:57.0", "29:57.0", "29:57.0", "29:57.1", "29:57.1", "29:57.1", "29:57.2", "29:57.2", "29:57.2", "29:57.3", "29:57.3", "29:57.3", "29:57.4", "29:57.4", "29:57.4", "29:57.5", "29:57.5", "29:57.5", "29:57.6", "29:57.6", "29:57.6", "29:57.7", "29:57.7", "29:57.7", "29:57.8", "29:57.8", "29:57.8", "29:57.9", "29:57.9", "29:57.9", "29:58.0", "29:58.0", "29:58.0", "29:58.1", "29:58.1", "29:58.1", "29:58.2", "29:58.2", "29:58.2", "29:58.3", "29:58.3", "29:58.3", "29:58.4", "29:58.4", "29:58.4", "29:58.5", "29:58.5", "29:58.5", "29:58.6", "29:58.6", "29:58.6", "29:58.7", "29:58.7", "29:58.7", "29:58.8", "29:58.8", "29:58.8", "29:58.9", "29:58.9", "29:58.9", "29:59.0", "29:59.0", "29:59.0", "29:59.1", "29:59.1", "29:59.1", "29:59.2", "29:59.2", "29:59.2", "29:59.3", "29:59.3", "29:59.3", "29:59.4", "29:59.4", "29:59.4", "29:59.5", "29:59.5", "29:59.5", "29:59.6", "29:59.6", "29:59.6", "29:59.7", "29:59.7", "29:59.7", "29:59.8", "29:59.8", "29:59.8", "29:59.9", "29:59.9", "29:59.9", "30:00.0", "30:00.0", "30:00.0", "30:00.1", "30:00.1", "30:00.1", "30:00.2", "30:00.2", "30:00.2", "30:00.3", "30:00.3", "30:00.3", "30:00.4", "30:00.4", "30:00.4", "30:00.5", "30:00.5", "30:00.5", "30:00.6", "30:00.6", "30:00.6", "30:00.7", "30:00.7", "30:00.7", "30:00.8", "30:00.8", "30:00.8", "30:00.9", "30:00.9", "30:00.9", "30:01.0", "30:01.0", "30:01.0", "30:01.1", "30:01.1", "30:01.1", "30:01.2", "30:01.2", "30:01.2", "30:01.3", "30:01.3", "30:01.3", "30:01.4", "30:01.4", "30:01.4", "30:01.5", "30:01.5", "30:01.5", "30:01.6", "30:01.6", "30:01.6", "30:01.7", "30:01.7", "30:01.7", "30:01.8", "30:01.8", "30:01.8", "30:01.9", "30:01.9", "30:01.9", "30:02.0", "30:02.0", "30:02.0", "30:02.1", "30:02.1", "30:02.1", "30:02.2", "30:02.2", "30:02.2", "30:02.3", "30:02.3", "30:02.3", "30:02.4", "30:02.4", "30:02.4", "30:02.5", "30:02.5", "30:02.5", "30:02.6", "30:02.6", "30:02.6", "30:02.7", "30:02.7", "30:02.7", "30:02.8", "30:02.8", "30:02.8", "30:02.9", "30:02.9", "30:02.9", "30:03.0", "30:03.0", "30:03.0", "30:03.1", "30:03.1", "30:03.1", "30:03.2", "30:03.2", "30:03.2", "30:03.3", "30:03.3", "30:03.3", "30:03.4", "30:03.4", "30:03.4", "30:03.5", "30:03.5", "30:03.5", "30:03.6", "30:03.6", "30:03.6", "30:03.7", "30:03.7", "30:03.7", "30:03.8", "30:03.8", "30:03.8", "30:03.9", "30:03.9", "30:03.9", "30:04.0", "30:04.0", "30:04.0", "30:04.1", "30:04.1", "30:04.1", "30:04.2", "30:04.2", "30:04.2", "30:04.3", "30:04.3", "30:04.3", "30:04.4", "30:04.4", "30:04.4", "30:04.5", "30:04.5", "30:04.5", "30:04.6", "30:04.6", "30:04.6", "30:04.7", "30:04.7", "30:04.7", "30:04.8", "30:04.8", "30:04.8", "30:04.9", "30:04.9", "30:04.9", "30:05.0", "30:05.0", "30:05.0", "30:05.1", "30:05.1", "30:05.1", "30:05.2", "30:05.2", "30:05.2", "30:05.3", "30:05.3", "30:05.3", "30:05.4", "30:05.4", "30:05.4", "30:05.5", "30:05.5", "30:05.5", "30:05.6", "30:05.6", "30:05.6", "30:05.7", "30:05.7", "30:05.7", "30:05.8", "30:05.8", "30:05.8", "30:05.9", "30:05.9", "30:05.9", "30:06.0", "30:06.0", "30:06.0", "30:06.1", "30:06.1", "30:06.1", "30:06.2", "30:06.2", "30:06.2", "30:06.3", "30:06.3", "30:06.3", "30:06.4", "30:06.4", "30:06.4", "30:06.5", "30:06.5", "30:06.5", "30:06.6", "30:06.6", "30:06.6", "30:06.7", "30:06.7", "30:06.7", "30:06.8", "30:06.8", "30:06.8", "30:06.9", "30:06.9", "30:06.9", "30:07.0", "30:07.0", "30:07.0", "30:07.1", "30:07.1", "30:07.1", "30:07.2", "30:07.2", "30:07.2", "30:07.3", "30:07.3", "30:07.3", "30:07.4", "30:07.4", "30:07.4", "30:07.5", "30:07.5", "30:07.5", "30:07.6", "30:07.6", "30:07.6", "30:07.7", "30:07.7", "30:07.7", "30:07.8", "30:07.8", "30:07.8", "30:07.9", "30:07.9", "30:07.9", "30:08.0", "30:08.0", "30:08.0", "30:08.1", "30:08.1", "30:08.1", "30:08.2", "30:08.2", "30:08.2", "30:08.3", "30:08.3", "30:08.3", "30:08.4", "30:08.4", "30:08.4", "30:08.5", "30:08.5", "30:08.5", "30:08.6", "30:08.6", "30:08.6", "30:08.7", "30:08.7", "30:08.7", "30:08.8", "30:08.8", "30:08.8", "30:08.9", "30:08.9", "30:08.9", "30:09.0", "30:09.0", "30:09.0", "30:09.1", "30:09.1", "30:09.1", "30:09.2", "30:09.2", "30:09.2", "30:09.3", "30:09.3", "30:09.3", "30:09.4", "30:09.4", "30:09.4", "30:09.5", "30:09.5", "30:09.5", "30:09.6", "30:09.6", "30:09.6", "30:09.7", "30:09.7", "30:09.7", "30:09.8", "30:09.8", "30:09.8", "30:09.9", "30:09.9", "30:09.9", "30:10.0", "30:10.0", "30:10.0", "30:10.1", "30:10.1", "30:10.1", "30:10.2", "30:10.2", "30:10.2", "30:10.3", "30:10.3", "30:10.3", "30:10.4", "30:10.4", "30:10.4", "30:10.5", "30:10.5", "30:10.5", "30:10.6", "30:10.6", "30:10.6", "30:10.7", "30:10.7", "30:10.7", "30:10.8", "30:10.8", "30:10.8", "30:10.9", "30:10.9", "30:10.9", "30:11.0", "30:11.0", "30:11.0", "30:11.1", "30:11.1", "30:11.1", "30:11.2", "30:11.2", "30:11.2", "30:11.3", "30:11.3", "30:11.3", "30:11.4", "30:11.4", "30:11.4", "30:11.5", "30:11.5", "30:11.5", "30:11.6", "30:11.6", "30:11.6", "30:11.7", "30:11.7", "30:11.7", "30:11.8", "30:11.8", "30:11.8", "30:11.9", "30:11.9", "30:11.9", "30:12.0", "30:12.0", "30:12.0", "30:12.1", "30:12.1", "30:12.1", "30:12.2", "30:12.2", "30:12.2", "30:12.3", "30:12.3", "30:12.3", "30:12.4", "30:12.4", "30:12.4", "30:12.5", "30:12.5", "30:12.5", "30:12.6", "30:12.6", "30:12.6", "30:12.7", "30:12.7", "30:12.7", "30:12.8", "30:12.8", "30:12.8", "30:12.9", "30:12.9", "30:12.9", "30:13.0", "30:13.0", "30:13.0", "30:13.1", "30:13.1", "30:13.1", "30:13.2", "30:13.2", "30:13.2", "30:13.3", "30:13.3", "30:13.3", "30:13.4", "30:13.4", "30:13.4", "30:13.5", "30:13.5", "30:13.5", "30:13.6", "30:13.6", "30:13.6", "30:13.7", "30:13.7", "30:13.7", "30:13.8", "30:13.8", "30:13.8", "30:13.9", "30:13.9", "30:13.9", "30:14.0", "30:14.0", "30:14.0", "30:14.1", "30:14.1", "30:14.1", "30:14.2", "30:14.2", "30:14.2", "30:14.3", "30:14.3", "30:14.3", "30:14.4", "30:14.4", "30:14.4", "30:14.5", "30:14.5", "30:14.5", "30:14.6", "30:14.6", "30:14.6", "30:14.7", "30:14.7", "30:14.7", "30:14.8", "30:14.8", "30:14.8", "30:14.9", "30:14.9", "30:14.9", "30:15.0", "30:15.0", "30:15.0", "30:15.1", "30:15.1", "30:15.1", "30:15.2", "30:15.2", "30:15.2", "30:15.3", "30:15.3", "30:15.3", "30:15.4", "30:15.4", "30:15.4", "30:15.5", "30:15.5", "30:15.5", "30:15.6", "30:15.6", "30:15.6", "30:15.7", "30:15.7", "30:15.7", "30:15.8", "30:15.8", "30:15.8", "30:15.9", "30:15.9", "30:15.9", "30:16.0", "30:16.0", "30:16.0", "30:16.1", "30:16.1", "30:16.1", "30:16.2", "30:16.2", "30:16.2", "30:16.3", "30:16.3", "30:16.3", "30:16.4", "30:16.4", "30:16.4", "30:16.5", "30:16.5", "30:16.5", "30:16.6", "30:16.6", "30:16.6", "30:16.7", "30:16.7", "30:16.7", "30:16.8", "30:16.8", "30:16.8", "30:16.9", "30:16.9", "30:16.9", "30:17.0", "30:17.0", "30:17.0", "30:17.1", "30:17.1", "30:17.1", "30:17.2", "30:17.2", "30:17.2", "30:17.3", "30:17.3", "30:17.3", "30:17.4", "30:17.4", "30:17.4", "30:17.5", "30:17.5", "30:17.5", "30:17.6", "30:17.6", "30:17.6", "30:17.7", "30:17.7", "30:17.7", "30:17.8", "30:17.8", "30:17.8", "30:17.9", "30:17.9", "30:17.9", "30:18.0", "30:18.0", "30:18.0", "30:18.1", "30:18.1", "30:18.1", "30:18.2", "30:18.2", "30:18.2", "30:18.3", "30:18.3", "30:18.3", "30:18.4", "30:18.4", "30:18.4", "30:18.5", "30:18.5", "30:18.5", "30:18.6", "30:18.6", "30:18.6", "30:18.7", "30:18.7", "30:18.7", "30:18.8", "30:18.8", "30:18.8", "30:18.9", "30:18.9", "30:18.9", "30:19.0", "30:19.0", "30:19.0", "30:19.1", "30:19.1", "30:19.1", "30:19.2", "30:19.2", "30:19.2", "30:19.3", "30:19.3", "30:19.3", "30:19.4", "30:19.4", "30:19.4", "30:19.5", "30:19.5", "30:19.5", "30:19.6", "30:19.6", "30:19.6", "30:19.7", "30:19.7", "30:19.7", "30:19.8", "30:19.8", "30:19.8", "30:19.9", "30:19.9", "30:19.9", "30:20.0", "30:20.0", "30:20.0", "30:20.1", "30:20.1", "30:20.1", "30:20.2", "30:20.2", "30:20.2", "30:20.3", "30:20.3", "30:20.3", "30:20.4", "30:20.4", "30:20.4", "30:20.5", "30:20.5", "30:20.5", "30:20.6", "30:20.6", "30:20.6", "30:20.7", "30:20.7", "30:20.7", "30:20.8", "30:20.8", "30:20.8", "30:20.9", "30:20.9", "30:20.9", "30:21.0", "30:21.0", "30:21.0", "30:21.1", "30:21.1", "30:21.1", "30:21.2", "30:21.2", "30:21.2", "30:21.3", "30:21.3", "30:21.3", "30:21.4", "30:21.4", "30:21.4", "30:21.5", "30:21.5", "30:21.5", "30:21.6", "30:21.6", "30:21.6", "30:21.7", "30:21.7", "30:21.7", "30:21.8", "30:21.8", "30:21.8", "30:21.9", "30:21.9", "30:21.9", "30:22.0", "30:22.0", "30:22.0", "30:22.1", "30:22.1", "30:22.1", "30:22.2", "30:22.2", "30:22.2", "30:22.3", "30:22.3", "30:22.3", "30:22.4", "30:22.4", "30:22.4", "30:22.5", "30:22.5", "30:22.5", "30:22.6", "30:22.6", "30:22.6", "30:22.7", "30:22.7", "30:22.7", "30:22.8", "30:22.8", "30:22.8", "30:22.9", "30:22.9", "30:22.9", "30:23.0", "30:23.0", "30:23.0", "30:23.1", "30:23.1", "30:23.1", "30:23.2", "30:23.2", "30:23.2", "30:23.3", "30:23.3", "30:23.3", "30:23.4", "30:23.4", "30:23.4", "30:23.5", "30:23.5", "30:23.5", "30:23.6", "30:23.6", "30:23.6", "30:23.7", "30:23.7", "30:23.7", "30:23.8", "30:23.8", "30:23.8", "30:23.9", "30:23.9", "30:23.9", "30:24.0", "30:24.0", "30:24.0", "30:24.1", "30:24.1", "30:24.1", "30:24.2", "30:24.2", "30:24.2", "30:24.3", "30:24.3", "30:24.3", "30:24.4", "30:24.4", "30:24.4", "30:24.5", "30:24.5", "30:24.5", "30:24.6", "30:24.6", "30:24.6", "30:24.7", "30:24.7", "30:24.7", "30:24.8", "30:24.8", "30:24.8", "30:24.9", "30:24.9", "30:24.9", "30:25.0", "30:25.0", "30:25.0", "30:25.1", "30:25.1", "30:25.1", "30:25.2", "30:25.2", "30:25.2", "30:25.3", "30:25.3", "30:25.3", "30:25.4", "30:25.4", "30:25.4", "30:25.5", "30:25.5", "30:25.5", "30:25.6", "30:25.6", "30:25.6", "30:25.7", "30:25.7", "30:25.7", "30:25.8", "30:25.8", "30:25.8", "30:25.9", "30:25.9", "30:25.9", "30:26.0", "30:26.0", "30:26.0", "30:26.1", "30:26.1", "30:26.1", "30:26.2", "30:26.2", "30:26.2", "30:26.3", "30:26.3", "30:26.3", "30:26.4", "30:26.4", "30:26.4", "30:26.5", "30:26.5", "30:26.5", "30:26.6", "30:26.6", "30:26.6", "30:26.7", "30:26.7", "30:26.7", "30:26.8", "30:26.8", "30:26.8", "30:26.9", "30:26.9", "30:26.9", "30:27.0", "30:27.0", "30:27.0", "30:27.1", "30:27.1", "30:27.1", "30:27.2", "30:27.2", "30:27.2", "30:27.3", "30:27.3", "30:27.3", "30:27.4", "30:27.4", "30:27.4", "30:27.5", "30:27.5", "30:27.5", "30:27.6", "30:27.6", "30:27.6", "30:27.7", "30:27.7", "30:27.7", "30:27.8", "30:27.8", "30:27.8", "30:27.9", "30:27.9", "30:27.9", "30:28.0", "30:28.0", "30:28.0", "30:28.1", "30:28.1", "30:28.1", "30:28.2", "30:28.2", "30:28.2", "30:28.3", "30:28.3", "30:28.3", "30:28.4", "30:28.4", "30:28.4", "30:28.5", "30:28.5", "30:28.5", "30:28.6", "30:28.6", "30:28.6", "30:28.7", "30:28.7", "30:28.7", "30:28.8", "30:28.8", "30:28.8", "30:28.9", "30:28.9", "30:28.9", "30:29.0", "30:29.0", "30:29.0", "30:29.1", "30:29.1", "30:29.1", "30:29.2", "30:29.2", "30:29.2", "30:29.3", "30:29.3", "30:29.3", "30:29.4", "30:29.4", "30:29.4", "30:29.5", "30:29.5", "30:29.5", "30:29.6", "30:29.6", "30:29.6", "30:29.7", "30:29.7", "30:29.7", "30:29.8", "30:29.8", "30:29.8", "30:29.9", "30:29.9", "30:29.9", "30:30.0", "30:30.0", "30:30.0", "30:30.1", "30:30.1", "30:30.1", "30:30.2", "30:30.2", "30:30.2", "30:30.3", "30:30.3", "30:30.3", "30:30.4", "30:30.4", "30:30.4", "30:30.5", "30:30.5", "30:30.5", "30:30.6", "30:30.6", "30:30.6", "30:30.7", "30:30.7", "30:30.7", "30:30.8", "30:30.8", "30:30.8", "30:30.9", "30:30.9", "30:30.9", "30:31.0", "30:31.0", "30:31.0", "30:31.1", "30:31.1", "30:31.1", "30:31.2", "30:31.2", "30:31.2", "30:31.3", "30:31.3", "30:31.3", "30:31.4", "30:31.4", "30:31.4", "30:31.5", "30:31.5", "30:31.5", "30:31.6", "30:31.6", "30:31.6", "30:31.7", "30:31.7", "30:31.7", "30:31.8", "30:31.8", "30:31.8", "30:31.9", "30:31.9", "30:31.9", "30:32.0", "30:32.0", "30:32.0", "30:32.1", "30:32.1", "30:32.1", "30:32.2", "30:32.2", "30:32.2", "30:32.3", "30:32.3", "30:32.3", "30:32.4", "30:32.4", "30:32.4", "30:32.5", "30:32.5", "30:32.5", "30:32.6", "30:32.6", "30:32.6", "30:32.7", "30:32.7", "30:32.7", "30:32.8", "30:32.8", "30:32.8", "30:32.9", "30:32.9", "30:32.9", "30:33.0", "30:33.0", "30:33.0", "30:33.1", "30:33.1", "30:33.1", "30:33.2", "30:33.2", "30:33.2", "30:33.3", "30:33.3", "30:33.3", "30:33.4", "30:33.4", "30:33.4", "30:33.5", "30:33.5", "30:33.5", "30:33.6", "30:33.6", "30:33.6", "30:33.7", "30:33.7", "30:33.7", "30:33.8", "30:33.8", "30:33.8", "30:33.9", "30:33.9", "30:33.9", "30:34.0", "30:34.0", "30:34.0", "30:34.1", "30:34.1", "30:34.1", "30:34.2", "30:34.2", "30:34.2", "30:34.3", "30:34.3", "30:34.3", "30:34.4", "30:34.4", "30:34.4", "30:34.5", "30:34.5", "30:34.5", "30:34.6", "30:34.6", "30:34.6", "30:34.7", "30:34.7", "30:34.7", "30:34.8", "30:34.8", "30:34.8", "30:34.9", "30:34.9", "30:34.9", "30:35.0", "30:35.0", "30:35.0", "30:35.1", "30:35.1", "30:35.1", "30:35.2", "30:35.2", "30:35.2", "30:35.3", "30:35.3", "30:35.3", "30:35.4", "30:35.4", "30:35.4", "30:35.5", "30:35.5", "30:35.5", "30:35.6", "30:35.6", "30:35.6", "30:35.7", "30:35.7", "30:35.7", "30:35.8", "30:35.8", "30:35.8", "30:35.9", "30:35.9", "30:35.9", "30:36.0", "30:36.0", "30:36.0", "30:36.1", "30:36.1", "30:36.1", "30:36.2", "30:36.2", "30:36.2", "30:36.3", "30:36.3", "30:36.3", "30:36.4", "30:36.4", "30:36.4", "30:36.5", "30:36.5", "30:36.5", "30:36.6", "30:36.6", "30:36.6", "30:36.7", "30:36.7", "30:36.7", "30:36.8", "30:36.8", "30:36.8", "30:36.9", "30:36.9", "30:36.9", "30:37.0", "30:37.0", "30:37.0", "30:37.1", "30:37.1", "30:37.1", "30:37.2", "30:37.2", "30:37.2", "30:37.3", "30:37.3", "30:37.3", "30:37.4", "30:37.4", "30:37.4", "30:37.5", "30:37.5", "30:37.5", "30:37.6", "30:37.6", "30:37.6", "30:37.7", "30:37.7", "30:37.7", "30:37.8", "30:37.8", "30:37.8", "30:37.9", "30:37.9", "30:37.9", "30:38.0", "30:38.0", "30:38.0", "30:38.1", "30:38.1", "30:38.1", "30:38.2", "30:38.2", "30:38.2", "30:38.3", "30:38.3", "30:38.3", "30:38.4", "30:38.4", "30:38.4", "30:38.5", "30:38.5", "30:38.5", "30:38.6", "30:38.6", "30:38.6", "30:38.7", "30:38.7", "30:38.7", "30:38.8", "30:38.8", "30:38.8", "30:38.9", "30:38.9", "30:38.9", "30:39.0", "30:39.0", "30:39.0", "30:39.1", "30:39.1", "30:39.1", "30:39.2", "30:39.2", "30:39.2", "30:39.3", "30:39.3", "30:39.3", "30:39.4", "30:39.4", "30:39.4", "30:39.5", "30:39.5", "30:39.5", "30:39.6", "30:39.6", "30:39.6", "30:39.7", "30:39.7", "30:39.7", "30:39.8", "30:39.8", "30:39.8", "30:39.9", "30:39.9", "30:39.9", "30:40.0", "30:40.0", "30:40.0", "30:40.1", "30:40.1", "30:40.1", "30:40.2", "30:40.2", "30:40.2", "30:40.3", "30:40.3", "30:40.3", "30:40.4", "30:40.4", "30:40.4", "30:40.5", "30:40.5", "30:40.5", "30:40.6", "30:40.6", "30:40.6", "30:40.7", "30:40.7", "30:40.7", "30:40.8", "30:40.8", "30:40.8", "30:40.9", "30:40.9", 
